vi "ESA-C Move Absolute v10.5.2.vi"(1 "Running":refnum<vi>, 3 "Drive New Abs. Positions":T1={"Drive X Set"=10.0, "Drive Y Set"=10.0, "Drive Z Set"=10.0} {"Drive X Set" min=10.0 max=160.0 step=0.1 format="%.1f"; "Drive Z Set" min=10.0 max=160.0 step=0.1 format="%.1f"; "Drive Y Set" min=10.0 max=160.0 step=0.1 format="%.1f"}, 4 "Drive Connection Settings":T2={"Objective GPIB-Port"=4, "Stage GPIB-Port"=4, "Drive Selector"=0, "Drive Velocity (V/s)"=5.0} {"Drive Velocity (V/s)" min=10.0 max=160.0 step=0.1 format="%.1f"; "Drive Selector" items=["Obj.", "Stage"]; "Stage GPIB-Port" min=1 max=20 step=1 format="%#.0f"; "Objective GPIB-Port" min=1 max=20 step=1 format="%#.0f"}) -> ()   [LabVIEW 2010]
uses:
  TypeDefs/ESA-C Connection Settings.ctl
  TypeDefs/ESA-C Set Positions.ctl
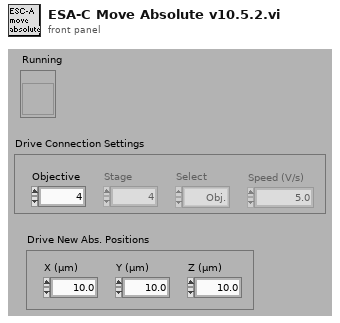
[diagram p1: front panel]
types:
  T1 = typedef "ESA-C Set Positions.ctl" = cluster{"Drive X Set":dbl, "Drive Y Set":dbl, "Drive Z Set":dbl}
  T2 = typedef "ESA-C Connection Settings.ctl" = cluster{"Objective GPIB-Port":i32, "Stage GPIB-Port":i32, "Drive Selector":u16, "Drive Velocity (V/s)":dbl}
  T3 = typedef "ESA-C Current Values.ctl" = cluster{"Voltages":cluster{"Drive X Voltage":dbl, "Drive Y Voltage":dbl, "Drive Z Voltage":dbl}, "Position":cluster{"Drive X Position":dbl, "Drive Y Position":dbl, "Drive Z Position":dbl}}
  T4 = cluster{"Drive X Voltage":dbl, "Drive Y Voltage":dbl, "Drive Z Voltage":dbl}
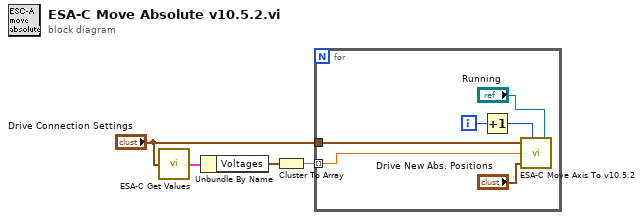
[diagram p0: block diagram]
diagram:
  n1 = call "ESA-C Get Values.vi"("Drive Connection Settings"="Drive Connection Settings") -> ("Drive Current Values"=w4:T3)
  n2 = Unbundle By Name(w4) -> ("Voltages"=w3:T4)
  n3 = Cluster To Array(cluster=w3) -> (array=w2:dbl[])
  n4 = for {
    tunnel: w2 -> [w8] mode=indexing
    tunnel: "Drive Connection Settings" -> [w7]
    i -> [w10]
    n5 = Increment(x=w10) -> (x+1=w9:i32)
    n6 = call "ESA-C Move Axis To v10.5.2.vi"("Drive Connection Settings"=w7, "Axis"=w9, "Current Voltage (V)"=w8, "Drive New Abs. Positions"="Drive New Abs. Positions", "Running"="Running") -> ()  [unwired: 2 in]
  }
